vi "read config.vi"(8 "error in (no error)":errorcluster, 10 "Path":path, 11 "Torque Transducer in":refnum<class "Torque Transducer.lvclass">) -> (0 "error out":errorcluster, 3 "Torque Transducer out":refnum<class "Torque Transducer.lvclass">)   [LabVIEW 2025, in "Torque Transducer.lvclass"]
uses:
  Torque Transducer.lvclass
  Torque Transducer.lvclass/Torque Transducer.ctl
  768bf59a-7fb3-48fc-a193-69b4e69d2ac8.vi
  <vilib>/JDP Science/JSONtext/JSON text to Variant.vi
  <vilib>/JDP Science/JSONtext/LVClass Serializer/JSONtext LVClass Serializer.lvclass
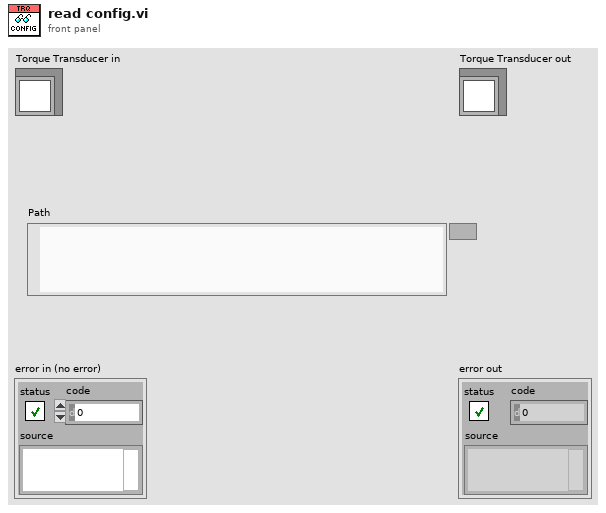
[diagram p1: front panel]
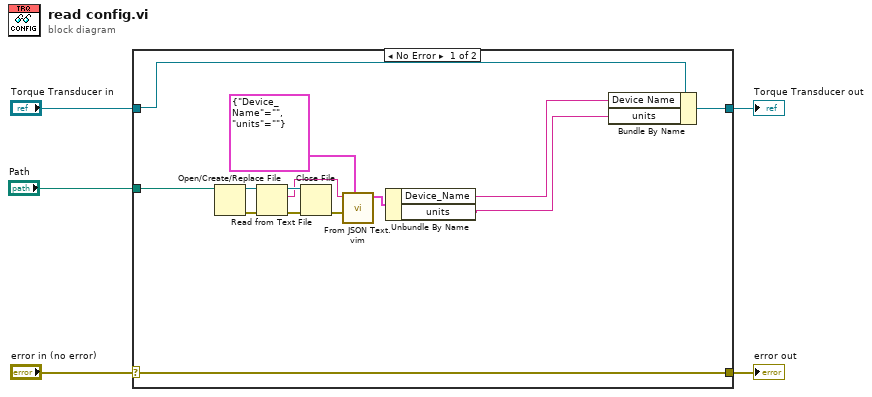
[diagram p0: block diagram]
diagram:
  n1 = case shown="No Error" "error in (no error)" {
    selector: "error in (no error)" -> [w19 w21]
    tunnel: [w19 w21] -> w4
    tunnel: [w18 w20] -> w2
    tunnel: "Torque Transducer in" -> [w17 w20]
    tunnel: "Path" -> [w8 _]
    frame No Error {
      n2 = Open/Create/Replace File(file path (use dialog)=w8) -> (refnum out=w13:refnum<file>, error out=w16:errorcluster)  [unwired: 5 in, 1 out]
      n3 = Read from Text File(file (use dialog)=w13, error in=w16) -> (refnum out=w14:refnum<file>, text=w12:string, error out=w15:errorcluster)  [unwired: 2 in, 1 out]
      n4 = Close File(refnum=w14, error in=w15) -> (error out=w11:errorcluster)  [unwired: 1 out]
      n5 = call "From JSON Text.vim"("Data Type and Default Value"=cluster{"Device_Name":string, "units":string} {"Device_Name"="", "units"=""}, "error in (no error)"=w11, "JSON"=w12) -> ("Data out"=w10:cluster{"Device_Name":string, "units":string})  [unwired: 7 in, 1 out]
      n6 = Unbundle By Name(w10) -> ("Device_Name"=w7:string, "units"=w6:string)
      n7 = Bundle By Name(cluster=w17, "Device Name"=w7, "units"=w6) -> (w18:refnum<class "Torque Transducer.lvclass">)
    }
    frame Error {
    }
  }
  "error out" <- w4
  "Torque Transducer out" <- w2
